vi "WaveformSimulator.vi"(10 "Waveform Parameters":T1, 11 "Digitizing Parameters":T2) -> (2 "XY Graph":cluster{"t":dbl[], "x":dbl[]}(graph))   [LabVIEW 2015]
uses:
  <vilib>/imath/engines/lvmath2/RunTimeEngine/Managers/WorkSpace/UID Generator.vi
  <vilib>/imath/engines/lvmath2/RunTimeEngine/RunTimeType/NIMS_RunTimeType_From StrictType (excl LVString).vi
  <instcachedir>/0/NIMS_RunTimeType_From StrictType (excl LVString)_EB1C38A9BC5048DA9ABDA8F781E54D21.lvgen/NIMS_RunTimeType_From StrictType (excl LVString)_EB1C38A9BC5048DA9ABDA8F781E54D21_000.vi
  <vilib>/imath/engines/lvmath2/RunTimeEngine/LocalVariableDefStatement/MC_LocalVariableDefStatement_Display.vi
  <vilib>/imath/engines/lvmath2/RunTimeEngine/RangeToken/NIMS_Range.vi
  <instcachedir>/0/NIMS_Range_D919CC09935940E88F755EC1C6F49AC1.lvgen/NIMS_Range_D919CC09935940E88F755EC1C6F49AC1_000.vi
  <vilib>/imathl/engines/lvmath/Functions/Error Handling/Create Error.vi
  <vilib>/imath/engines/lvmath2/RunTimeEngine/ArithmeticOperatorToken/NIMS_ArithmeticOperator_plus.vi
  <instcachedir>/0/NIMS_ArithmeticOperator_plus_A4F2756F5ADB4A0090E0DBD7C10701C8.lvgen/NIMS_ArithmeticOperator_plus_A4F2756F5ADB4A0090E0DBD7C10701C8_004.vi
  <vilib>/imath/engines/lvmath2/RunTimeEngine/BuiltInFunctions/gensignal/NIMS_gensignal(str,RS,RS,RS).vi
  <vilib>/imath/engines/lvmath2/RunTimeEngine/BuiltInFunctions/linramp/NIMS_linramp.vi
  <vilib>/imath/engines/lvmath2/RunTimeEngine/VariableToken/NIMS_VariableToken_CondDefined.vi
  <instcachedir>/0/NIMS_VariableToken_CondDefined_FE30D0A1BFB24F098D41DEBABFE96BE1.lvgen/NIMS_VariableToken_CondDefined_FE30D0A1BFB24F098D41DEBABFE96BE1_001.vi
  <vilib>/imath/engines/lvmath2/RunTimeEngine/NodeEndStatement/NIMS_NodeEndStatement_Get Vector.vi
  <instcachedir>/0/NIMS_NodeEndStatement_Get Vector_ED7FC4F6B50246F79D573C75B2E51AF8.lvgen/NIMS_NodeEndStatement_Get Vector_ED7FC4F6B50246F79D573C75B2E51AF8_001.vi
  <vilib>/imath/engines/lvmath/Functions/Error Handling/MergeErrorsWrapper.vi
  <vilib>/imath/engines/lvmath2/RunTimeEngine/Managers/SymbolTable/Clear UID.vi
  <vilib>/imath/engines/lvmath2/RunTimeEngine/NodeEndStatement/NIMS_NodeEndStatement_Output.vi
  <instcachedir>/0/NIMS_NodeEndStatement_Output_53EC0D466D134D7ABD903AC30B43404B.lvgen/NIMS_NodeEndStatement_Output_53EC0D466D134D7ABD903AC30B43404B_005.vi
  <vilib>/imath/engines/lvmath2/RunTimeEngine/ErrorHandling/NIMS_Finalize Error.vi
  <vilib>/imath/engines/lvmath2/RunTimeEngine/Managers/SymbolTable/NIMS_WorkSpace.lvlib
panel:
  out "x":dbl[](array[numeric])
  out "Time":dbl[](array[numeric])
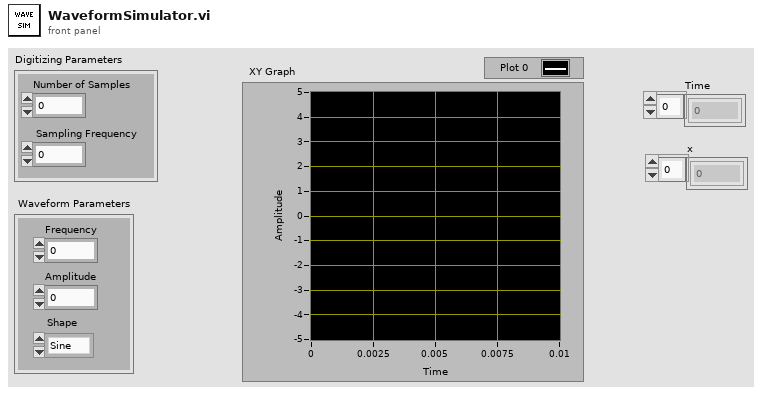
[diagram p1: front panel]
types:
  T1 = cluster{"Frequency":dbl, "Amplitude":dbl, "Shape":enum16{"Sine", "Cosine", "DC Level", "Square", "User-Defined"}}
  T2 = cluster{"Number of Samples":dbl, " Sampling Frequency":dbl}
  T3 = enum16{"Sine", "Cosine", "DC Level", "Square", "User-Defined"}
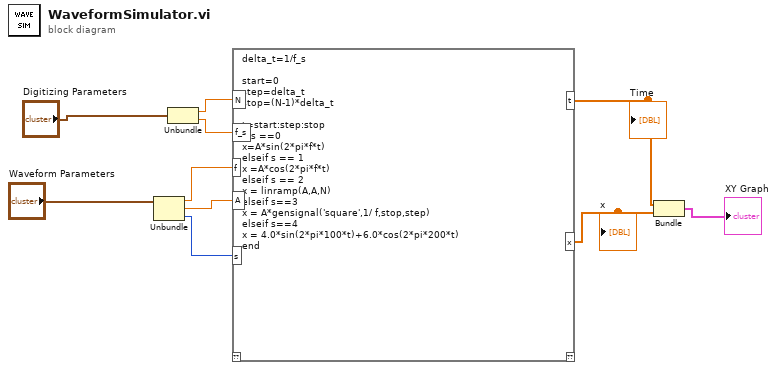
[diagram p0: block diagram]
diagram:
  n1 = Unbundle("Waveform Parameters") -> ("Frequency"=w4:dbl, "Amplitude"=w3:dbl, "Shape"=w1:T3)
  n2 = Unbundle("Digitizing Parameters") -> ("Number of Samples"=w7:dbl, "Sampling Frequency"=w6:dbl)
  n3 = mathscript code="delta_t=1/f_s\n\nstart=0\nstep=delta_t\nstop=(N-1)*delta_t\n\nt=start:step:stop\nif s ==0\nx=A*sin(2*pi*f*t)\nelseif s == 1\nx =A*cos(2*pi*f*t)\nelseif s == 2\nx = linramp(A,A,N)\nelseif s==3\nx = A*gensignal('square',1/ f,stop,step)\nelseif s==4\nx = 4.0*sin(2*pi*100*t)+6.0*cos(2*pi*200*t)\nend"("N"=w7, "f_s"=w6, "f"=w4, "A"=w3, "s"=w1) -> ("t"=w9:dbl[], "x"=w10:dbl[])  [unwired: 1 in, 1 out]
  "Time" <- w9
  "x" <- w10
  n4 = Bundle("t"=w9, "x"=w10) -> (→"XY Graph":cluster{"t":dbl[], "x":dbl[]})  [unwired: 1 in]
